vi "Process Secondary.vi"(11 "Arilou in":refnum<class "Arilou.lvclass">) -> (2 "New Elements":refnum<class "Element.lvclass">[](array[class]), 3 "Arilou out":refnum<class "Arilou.lvclass">)   [LabVIEW 2021, in "Arilou.lvclass"]
uses:
  Arilou.lvclass
  C:/dev/LabVIEW/LabMelee/Source/Application Specific/Element/Element.lvclass
  Element/Element.lvclass
  Element/Element.lvclass/Element.ctl
  Re-use Libraries/Vector 2D/Vector 2D.lvclass/Vector 2D.ctl
  Motion/Motion.lvclass/Motion.ctl
  <vilib>/numeric/Random Number (Range) DBL.vi
  Re-use Libraries/Vector 2D/Vector 2D.lvclass
  Motion/Motion.lvclass
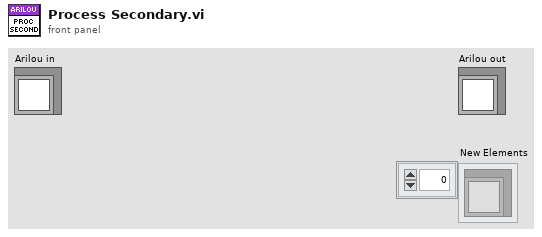
[diagram p1: front panel]
types:
  T1 = typedef "Constants.ctl" = cluster{"Colours":cluster{"OK":u32, "Warning":u32, "Error":u32, "Red":u32, "Green":u32, "Blue":u32, "Yellow":u32}, "System":cluster{"Target Frames Second":dbl, "Windows Size":refnum<class "Vector 2D.lvclass">, "World Size":refnum<class "Vector 2D.lvclass">, "Battle Area Size":refnum<class "Vector 2D.lvclass">, "Sidebar Width":sgl, "SC2 Frame Rate [Seconds/Frame]":sgl, "Sidebar Player 2 Y Offset":sgl}, "Game":cluster{"Maximum Asteroids":i32, "Max Energy":i32, "Max Crew":i32, "Maximum Stars":i32}}
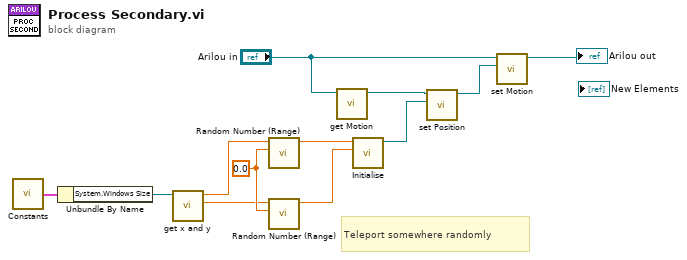
[diagram p0: block diagram]
diagram:
  w7 = 0.0 ("Low")
  # "Teleport somewhere randomly"
  n1 = call "Constants.vi"() -> ("Constants"=w4:T1)
  n2 = Unbundle By Name(w4) -> ("System.Windows Size"=w3:refnum<class "Vector 2D.lvclass">)
  n3 = call "get x and y.vi"("Vector 2D in"=w3) -> ("y"=w1:sgl, "x"=w2:sgl)  [unwired: 9 in]
  n4 = call-poly <vilib>:"Random Number (Range).vi"("lower bound (0)"=w7, "upper bound (100)"=w2) -> ("number"=w6:dbl)  [unwired: 9 in]
  n5 = call-poly <vilib>:"Random Number (Range).vi"("lower bound (0)"=w7, "upper bound (100)"=w1) -> ("number"=w5:dbl)  [unwired: 9 in]
  n6 = call "get Motion.vi"("Element in"="Arilou in") -> ("Motion"=w12:refnum<class "Motion.lvclass">)  [unwired: 10 in]
  n7 = call "Initialise.vi"("y"=w5, "x"=w6) -> ("Vector 2D out"=w8:refnum<class "Vector 2D.lvclass">)  [unwired: 9 in]
  n8 = call "set Position.vi"("Position"=w8, "Motion in"=w12) -> ("Motion out"=w11:refnum<class "Motion.lvclass">)  [unwired: 9 in]
  n9 = call "set Motion.vi"("Motion"=w11, "Element in"="Arilou in") -> ("Element out"=→"Arilou out":refnum<class "Arilou.lvclass">)  [unwired: 9 in]
